vi "WS1050_VSA_Convert_Data.vi"(6 "VSA_C3":string[][](array[string]), 8 "error in (no error)":errorcluster, 9 "VSA_C2":string[][](array[string]), 10 "VSA_C1":string[][](array[string]), 11 "Voltage":string[][](array[string])) -> (0 "error out":errorcluster, 1 "VSA_V3":string[][](array[string]), 2 "VSA_V2":string[][](array[string]), 3 "VSA_V1":string[][](array[string]))   [LabVIEW 2012]
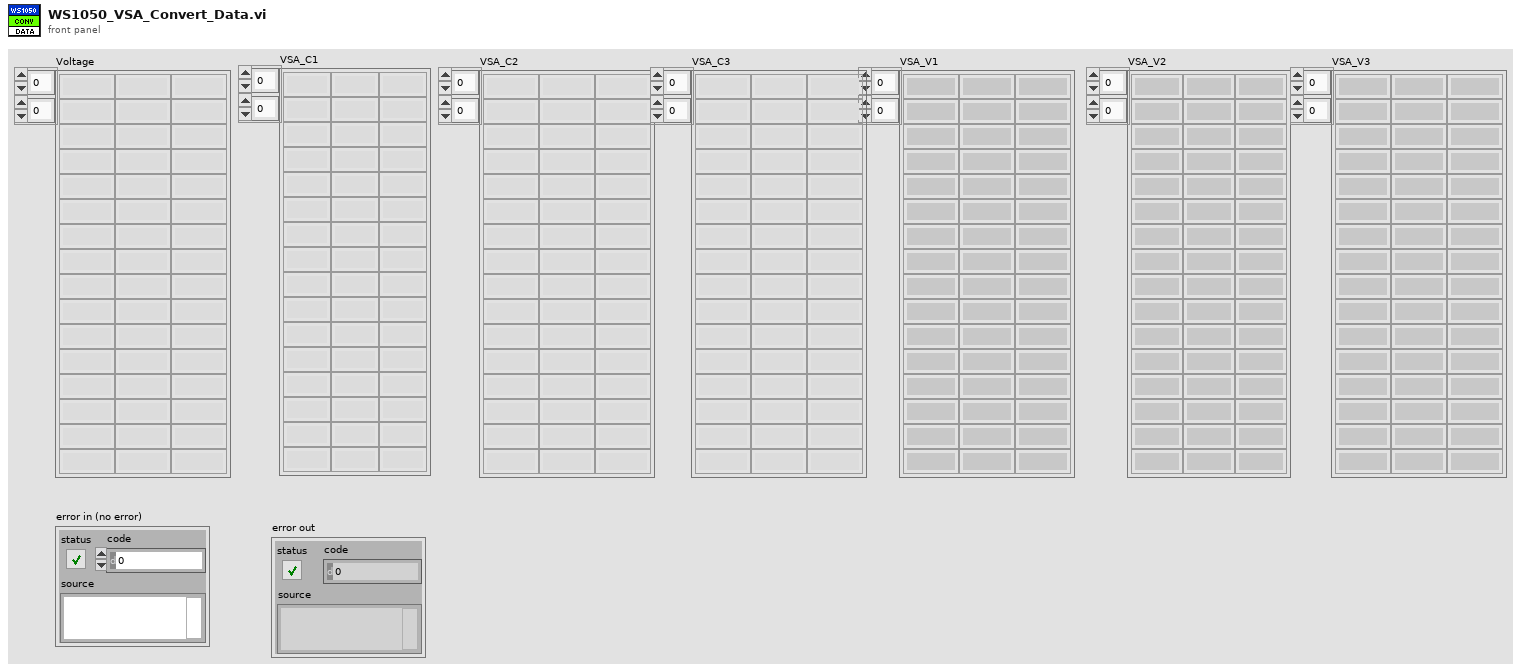
[diagram p1: front panel]
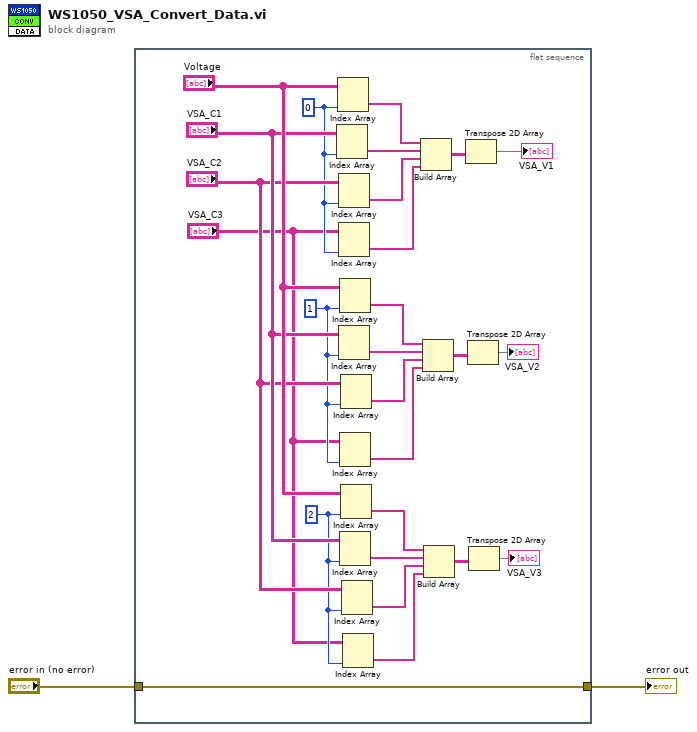
[diagram p0: block diagram]
diagram:
  n1 = flat-sequence {
    tunnel: "error in (no error)" -> [w3]
    tunnel: [w3] -> w1
    frame #0 {
      w6 = 2 ("disabled index (col)")
      w8 = 1 ("disabled index (col)")
      w10 = 0 ("disabled index (col)")
      n2 = Index Array(array="VSA_C1", index (col)=w10) -> (element=w27:string[])  [unwired: 1 in]
      n3 = Index Array(array="Voltage", index (col)=w10) -> (element=w28:string[])  [unwired: 1 in]
      n4 = Index Array(array="VSA_C2", index (col)=w10) -> (element=w26:string[])  [unwired: 1 in]
      n5 = Index Array(array="VSA_C3", index (col)=w10) -> (element=w9:string[])  [unwired: 1 in]
      n6 = Index Array(array="VSA_C1", index (col)=w8) -> (element=w21:string[])  [unwired: 1 in]
      n7 = Index Array(array="Voltage", index (col)=w8) -> (element=w20:string[])  [unwired: 1 in]
      n8 = Index Array(array="VSA_C3", index (col)=w8) -> (element=w7:string[])  [unwired: 1 in]
      n9 = Index Array(array="VSA_C1", index (col)=w6) -> (element=w18:string[])  [unwired: 1 in]
      n10 = Index Array(array="VSA_C2", index (col)=w8) -> (element=w22:string[])  [unwired: 1 in]
      n11 = Index Array(array="Voltage", index (col)=w6) -> (element=w19:string[])  [unwired: 1 in]
      n12 = Index Array(array="VSA_C2", index (col)=w6) -> (element=w17:string[])  [unwired: 1 in]
      n13 = Index Array(array="VSA_C3", index (col)=w6) -> (element=w4:string[])  [unwired: 1 in]
      n14 = Build Array(w28, w27, w26, w9) -> (w25:string[][])
      n15 = Build Array(w20, w21, w22, w7) -> (w23:string[][])
      n16 = Build Array(w19, w18, w17, w4) -> (w16:string[][])
      n17 = Transpose 2D Array(2D array=w25) -> (transposed array=→"VSA_V1":string[][])
      n18 = Transpose 2D Array(2D array=w23) -> (transposed array=→"VSA_V2":string[][])
      n19 = Transpose 2D Array(2D array=w16) -> (transposed array=→"VSA_V3":string[][])
    }
  }
  "error out" <- w1
